vi "Create Event Type-Def for API Call.vi"(8 "error in (no error)":errorcluster, 11 "Control Path in":path) -> (0 "error out":errorcluster, 3 "Control Path out":path)   [LabVIEW 2018, in "Scripting.lvlib"]
uses:
  Scripting.lvlib
  Locale-Strings.ctl
  <vilib>/Utility/traverseref.llb/TRef TravTarget.ctl
  <vilib>/Utility/traverseref.llb/VI Scripting - Traverse.lvlib
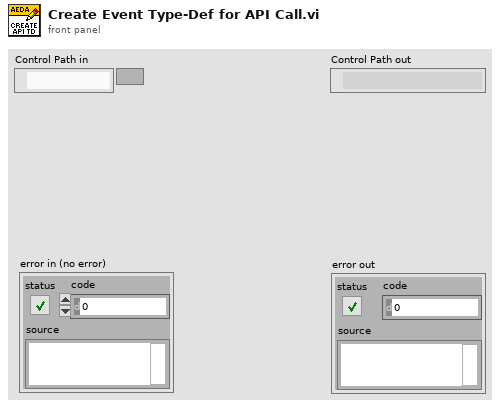
[diagram p1: front panel]
types:
  T1 = enum32{"Invalid", "Standard", "Closed", "Hidden", "Minimized", "Maximized"}
  T2 = typedef "TRef TravTarget.ctl" = enum16{"FP", "BD", "Other"}
  T3 = typedef "Scripting.lvlib/Locale-Strings.ctl" = enum16{"Event-Type-Def-Creation-API-Call"}
  T4 = enum32{"invalid VI type", "Standard VI", "Control VI", "Global VI", "Polymorphic VI", "Configuration VI", "SubSystem", "Facade VI", "Method VI", "Statechart Diagram VI"}
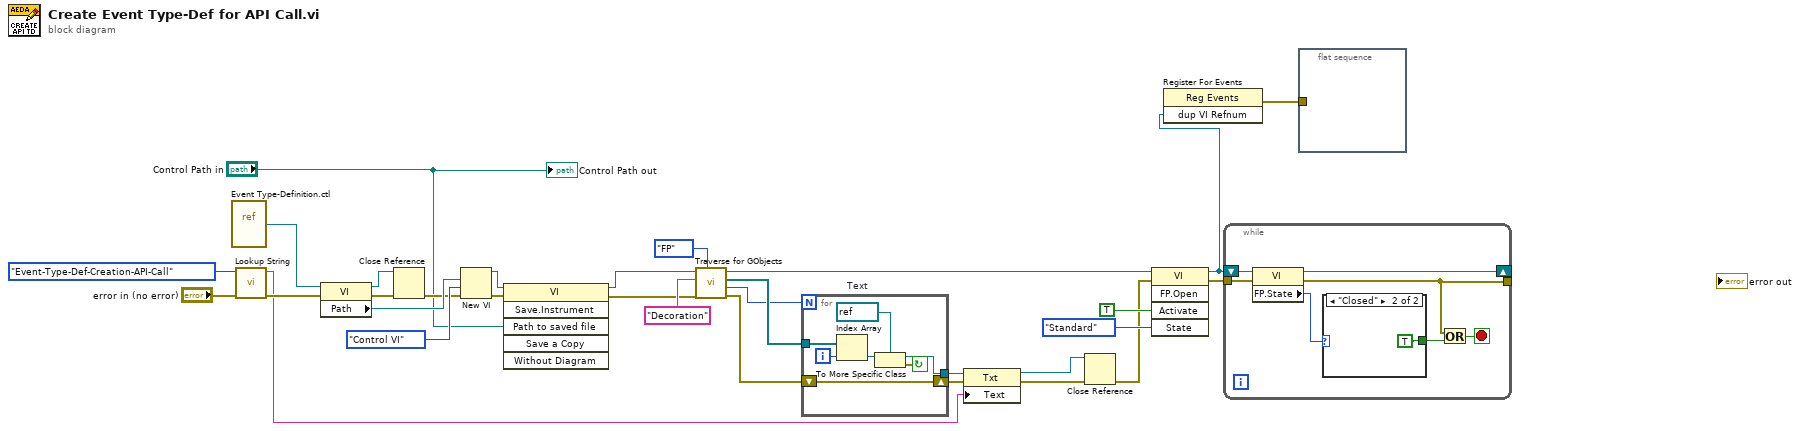
[diagram p0: block diagram]
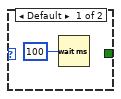
[diagram p2: hidden frame]
diagram:
  n1 = vi-ref "Event Type-Definition.ctl"() -> (w30:refnum<vi>)
  n2 = call "Lookup String.vi"("error in (no error)"="error in (no error)", "Locale String"=Locale-Strings."Event-Type-Def-Creation-API-Call") -> ("error out"=w24:errorcluster, "String"=w16:string)  [unwired: 8 in]
  n3 = property class="VI"(reference=w30, error in=w24) -> (reference out=w26:refnum<vi>, error out=w28:errorcluster, "Path"=w29:path)
  n4 = Close Reference(reference=w26, error in (no error)=w28) -> (error out=w27:errorcluster)
  n5 = New VI(8:w27, 9:T4."Control VI" ("vi type (standard vi)"), 10:w29) -> (0:w7:errorcluster, 3:w6:refnum<vi>)  [unwired: 4 in]
  n6 = invoke class="VI" method="Save.Instrument"(reference=w6, error in=w7, "Path to saved file"="Control Path in") -> (reference out=w4:refnum<vi>, error out=w5:errorcluster)  [unwired: 3 in, 4 out]
  n7 = call <vilib>:"Traverse for GObjects.vi"("Traverse Target"=TRef_TravTarget."FP", "error in (no error)"=w5, "Class Name"="Decoration", "VI Refnum"=w4) -> ("error out"=w19:errorcluster, "# of Refs"=w8:i32, "References"=w20:refnum<vi>[], "dup VI Refnum"=w3:refnum<vi>)  [unwired: 4 in]
  n8 = for {
    N: w8 -> [_]
    tunnel: w20 -> [w36]
    tunnel: [w38] -> w17
    shift-right: [w32] -> w18
    shift-left: w19 -> [w32]
    i -> [w33]
    stop <- w35 continue-if-true
    w37 = refnum<vi> refnum  # Text
    n9 = Index Array(array=w36, index=w33) -> (element=w34:refnum<vi>)
    n10 = To More Specific Class(target class=w37, reference=w34) -> (specific class reference=w38:refnum<vi>, error out=w35:errorcluster)  [unwired: 1 in]
  }
  n11 = property class="Txt"(reference=w17, error in=w18, "Text"=w16) -> (reference out=w11:refnum<vi>, error out=w12:errorcluster)
  n12 = Close Reference(reference=w11, error in (no error)=w12) -> (error out=w10:errorcluster)
  n13 = invoke class="VI" method="FP.Open"(reference=w3, error in=w10, "Activate"=TRUE ("Activate?"), "State"=T1."Standard") -> (reference out=w1:refnum<vi>, error out=w13:errorcluster)  [unwired: 1 in, 3 out]
  n14 = register-events(w1) -> (error out=w2:errorcluster)  [unwired: 2 in, 1 out]
  n15 = while {
    tunnel: w13 -> [w44]
    shift-right: [w41] -> _
    shift-left: w1 -> [w45]
    tunnel: [w39] -> _
    stop <- w40 stop-if-true
    n16 = property class="VI"(reference=w45, error in=w44) -> (reference out=w41:refnum<vi>, error out=w39:errorcluster, "FP.State"=w43:T1)
    n17 = case shown="\"Closed\"" w43 {
      tunnel: [_ TRUE] -> w42
      frame Default {
        n18 = Wait (ms)(milliseconds to wait=u32 100) -> ()  [unwired: 1 out]
      }
      frame "Closed" {
      }
    }
    n19 = Or(x=w39, y=w42) -> (x .or. y?=w40:bool)
  }
  n20 = flat-sequence {
    tunnel: w2 -> [_]
    frame #0 {
    }
  }
  "Control Path out" <- "Control Path in"
